vi "AlliGator Get tau1, tau2 & a1.vi"(10 "Best Fit Parameters":dbl[](array[numeric])) -> (0 "a 1":dbl, 1 "tau 2":dbl, 2 "tau 1":dbl)   [LabVIEW 2021, in "AlliGator Fit Method Benchmark.lvlib"]
doc: "Outputs tau1, tau2 and a1."
uses:
  AlliGator Fit Method Benchmark.lvlib
panel:
  # "see the AlliGator License on the block diagram (Ctrl+E or Window:Show Block Diagram)"
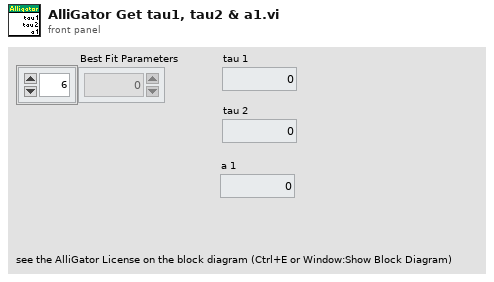
[diagram p1: front panel]
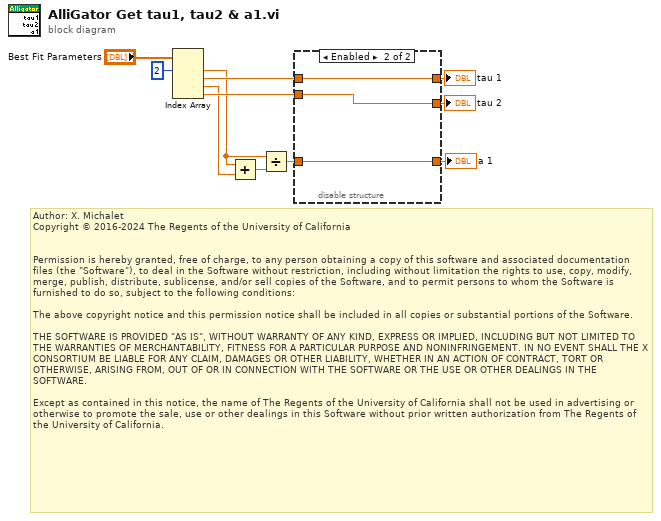
[diagram p0: block diagram]
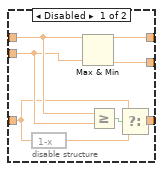
[diagram p2: hidden frame]
diagram:
  # "Author: X. Michalet\nCopyright © 2016-2024 The Regents of the University of California\n \n\nPermission is hereby granted, free of charge, to any person obtaining a copy of this software and associated documentation files (the \"Software\"), to deal in the Software without restriction, including without limitation the rights to use, copy, modify, merge, publish, distribute, sublicense, and/or sell copies of the Software, and to permit persons to whom the Software is furnished to do so, subject to the following conditions:\n\nThe above copyright notice and this permission notice shall be included in all copies or substantial portions of the Software.\n\nTHE SOFTWARE IS PROVIDED \"AS IS\", WITHOUT WARRANTY OF ANY KIND, EXPRESS OR IMPLIED, INCLUDING BUT NOT LIMITED TO THE WARRANTIES OF MERCHANTABILITY, FITNESS FOR A PARTICULAR PURPOSE AND NONINFRINGEMENT. IN NO EVENT SHALL THE X CONSORTIUM BE LIABLE FOR ANY CLAIM, DAMAGES OR OTHER LIABILITY, WHETHER IN AN ACTION OF CONTRACT, TORT OR OTHERWISE, ARISING FROM, OUT OF OR IN CONNECTION WITH THE SOFTWARE OR THE USE OR OTHER DEALINGS IN THE SOFTWARE.\n\nExcept as contained in this notice, the name of The Regents of the University of California shall not be used in advertising or otherwise to promote the sale, use or other dealings in this Software without prior written authorization from The Regents of the University of California."
  n1 = Index Array(array="Best Fit Parameters", index #1=2 ("index")) -> (element #1=w1:dbl, element #2=w7:dbl, element #3=w4:dbl, element #4=w6:dbl)  [unwired: 3 in]
  n2 = Add(x=w1, y=w4) -> (x+y=w3:dbl)
  n3 = Divide(x=w1, y=w3) -> (x/y=w2:dbl)
  n4 = disable-structure shown="Enabled" {
    disable-tunnel: [w19 w21] -> w11
    disable-tunnel: [w18 w22] -> w10
    disable-tunnel: w7 -> [w17 w22]
    disable-tunnel: w6 -> [w16 w21]
    disable-tunnel: [w15 w20] -> w5
    disable-tunnel: w2 -> [w14 w20]
    frame Disabled {
      n5 = expression code="1-x"(w14) -> (w12:dbl)
      n6 = Max & Min(x=w17, y=w16) -> (max(x,y)=w18:dbl, min(x,y)=w19:dbl)
      n7 = Greater Or Equal?(x=w17, y=w16) -> (x >= y?=w13:bool)
      n8 = Select(t=w14, s=w13, f=w12) -> (s? t:f=w15:dbl)
    }
    frame Enabled {
    }
  }
  "a 1" <- w5
  "tau 2" <- w11
  "tau 1" <- w10
